vi "front_panel_new.vi"() -> ()   [LabVIEW 2026]
uses:
  <vilib>/userDefined/High Color/IMAQdx.ctl
  <vilib>/vision/driver/NI_Vision_Acquisition_Software.lvlib
  <resource>/objmgr/imaqdx.rc
panel:
  in  "Space":bool
  in  "Ready to Speak":bool
  in  "Speak":bool
  out "Text":string
  in  "Hand":bool
  in  "Next_letter":bool
  in  "Input":bool
  in  "Filename":string
  out "Image":T1(plugin-control)
  out "Prediction":string
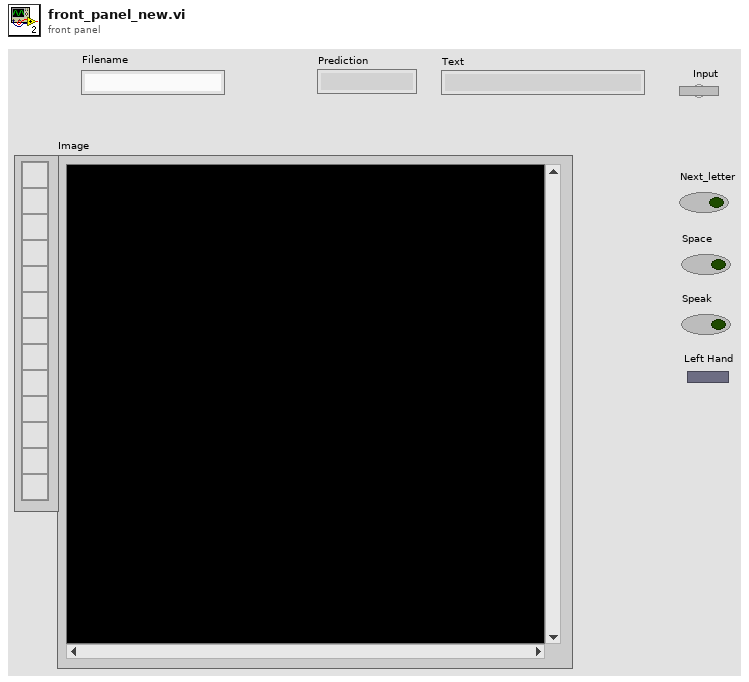
[diagram p1: front panel]
types:
  T1 = typedef "IMAQ Image.ctl" = refnum<image>
  T2 = typedef "IMAQdx.ctl" = refnum<k21>
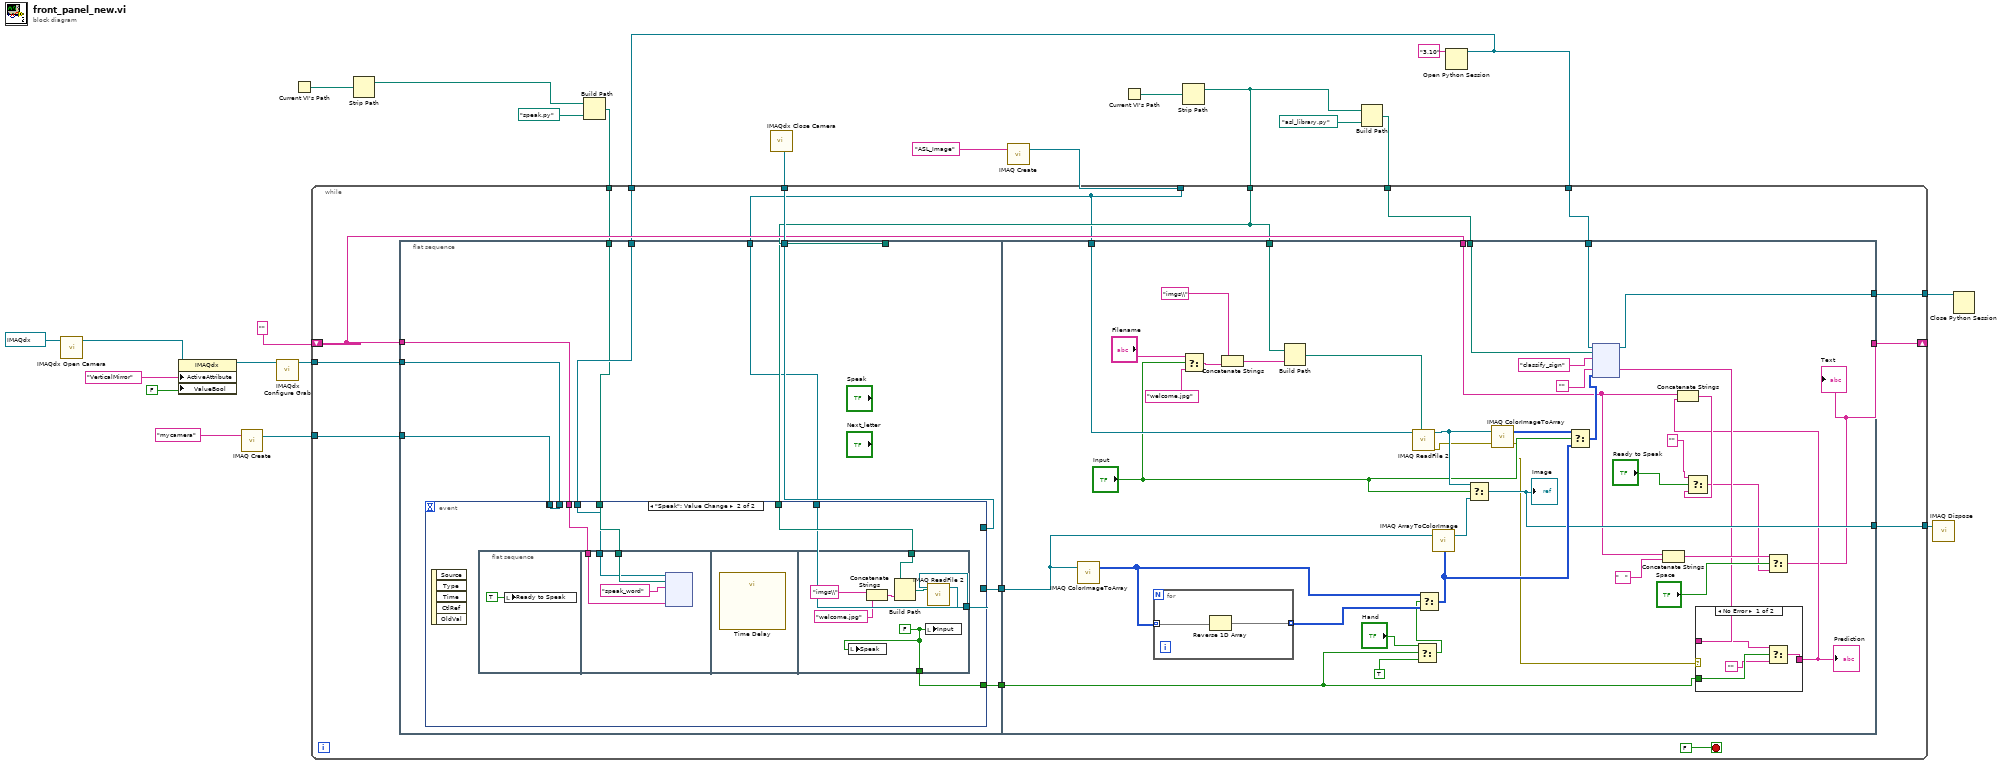
[diagram p0: block diagram]
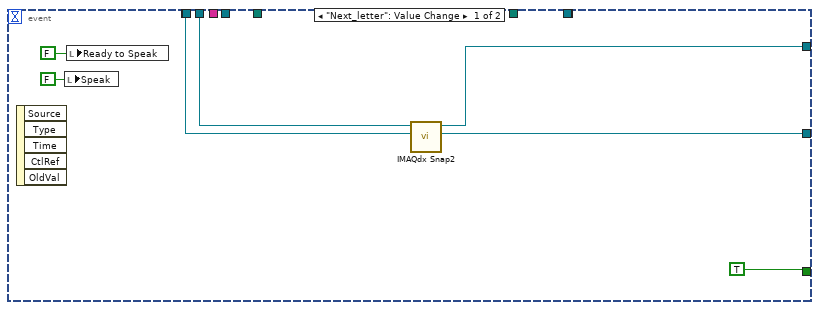
[diagram p2: hidden frame]
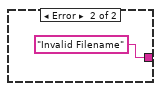
[diagram p3: hidden frame]
diagram:
  n1 = call <vilib>:"IMAQdx Open Camera.vi"("Session In"=T2 "cam0") -> ("Session Out"=w23:T2)  [unwired: 9 in, 1 out]
  n2 = property class="IMAQdx"(reference=w23, "ActiveAttribute"="VerticalMirror", "ValueBool"=FALSE) -> (reference out=w24:T2)  [unwired: 1 in, 1 out]
  n3 = call "IMAQ Create"("Image Name"="mycamera") -> ("New Image"=w17:T1)  [unwired: 4 in, 1 out]
  n4 = call <vilib>:"IMAQdx Configure Grab.vi"("Session In"=w24) -> ("Session Out"=w19:T2)  [unwired: 9 in, 1 out]
  n5 = Current VI's Path() -> (path=w4:path)
  n6 = Strip Path(path=w4) -> (stripped path=w2:path)  [unwired: 1 out]
  n7 = Build Path(base path=w2, name or relative path=path "speak.py" ("module path")) -> (appended path=w1:path)
  n8 = call "IMAQ Create"("Image Name"="ASL_Image") -> ("New Image"=w7:T1)  [unwired: 4 in, 1 out]
  n9 = Current VI's Path() -> (path=w12:path)
  n10 = Strip Path(path=w12) -> (stripped path=w9:path)  [unwired: 1 out]
  n11 = Build Path(base path=w9, name or relative path=path "asl_library.py" ("module path")) -> (appended path=w10:path)
  n12 = Open Python Session(python version="3.10" ("Python version")) -> (session out=w5:refnum<k35>)  [unwired: 2 in, 1 out]
  n13 = while {
    tunnel: w19 -> [w39]
    tunnel: w17 -> [w38]
    tunnel: [w37] -> w16
    tunnel: [w36] -> w15
    tunnel: [w35] -> w14
    tunnel: w5 -> [w34]
    tunnel: w10 -> [w33]
    tunnel: w9 -> [w28]
    tunnel: w7 -> [w27]
    shift-right: [w31] -> _
    shift-left: "" -> [w30]
    tunnel: w5 -> [w29]
    tunnel: w1 -> [w26]
    stop <- FALSE stop-if-true
    n14 = flat-sequence {
      tunnel: [w50] -> w40
      tunnel: w39 -> [w49]
      tunnel: w38 -> [w48]
      tunnel: [w47] -> w35
      tunnel: w30 -> [w46]
      tunnel: w29 -> [w45]
      tunnel: w28 -> [w44]
      tunnel: w27 -> [w43]
      tunnel: w26 -> [w42]
      tunnel: [w41] -> w25
      tunnel: w40 -> [w114]
      tunnel: [w106] -> w37
      tunnel: [w105] -> w36
      tunnel: w34 -> [w104]
      tunnel: w33 -> [w103]
      tunnel: w28 -> [w102]
      tunnel: w27 -> [w101]
      tunnel: w30 -> [w94]
      tunnel: [w83] -> w31
      tunnel: w25 -> [w86]
      frame #0 {
        n15 = event shown="[1] \"Speak\": Value Change" {
          selector: _ -> [_ _]
          dyn-events: _ -> [_ _]
          timeout: _ -> [_ _]
          tunnel: [w58 w62] -> w50
          tunnel: [w57 _] -> w47
          tunnel: w49 -> [w56 w66]
          tunnel: w48 -> [w55 _]
          tunnel: w46 -> [_ w60]
          tunnel: [_ w66] -> _
          tunnel: w45 -> [_ w61]
          tunnel: w44 -> [_ w64]
          tunnel: w43 -> [w52 w63]
          tunnel: w42 -> [_ w65]
          tunnel: [w52 _] -> _
          tunnel: [TRUE ("Input") w59] -> w41
          event "Next_letter": Value Change {
            n16 = event-data() -> ()  [unwired: 1 in, 5 out]
            n17 = local write "Speak"(FALSE ("Speak")) -> ()
            n18 = local write "Ready to Speak"(FALSE ("Ready_to_Speak")) -> ()
            n19 = call <vilib>:"IMAQdx Snap2.vi"("Image In"=w55, "Session In"=w56) -> ("Image Out"=w58:T1, "Session Out"=w57:T2)  [unwired: 7 in, 1 out]
          }
          event "Speak": Value Change {
            n20 = event-data() -> ()  [unwired: 1 in, 5 out]
            n21 = flat-sequence {
              tunnel: w65 -> [w71]
              tunnel: w60 -> [w69]
              tunnel: w61 -> [w68]
              tunnel: w64 -> [w75]
              tunnel: w63 -> [w74]
              tunnel: [w73] -> w62
              tunnel: [w72] -> w59
              frame #0 {
                n22 = local write "Ready to Speak"(TRUE ("Ready_to_Speak")) -> ()
              }
              frame #1 {
                n23 = node(w68, w71, "speak_word" ("function name"), w69) -> ()  [unwired: 4 in, 4 out]
              }
              frame #2 {
                n24 = call "Time Delay"() -> ()  [unwired: 11 in, 1 out]
              }
              frame #3 {
                w72 = FALSE ("Input")
                n25 = local write "Speak"(w72) -> ()
                n26 = Concatenate Strings("imgs\\" ("string"), "welcome.jpg" ("string")) -> (w78:string)
                n27 = Build Path(base path=w75, name or relative path=w78) -> (appended path=w79:path)
                n28 = local write "Input"(w72) -> ()
                n29 = call "IMAQ ReadFile 2"("File Path"=w79, "Image"=w74) -> ("Image Out"=w73:T1)  [unwired: 5 in, 4 out]
              }
            }
          }
        }
      }
      frame #1 {
        n30 = call "IMAQ ColorImageToArray"("Image"=w114) -> ("Image Pixels (U32)"=w108:u32[][])  [unwired: 3 in, 2 out]
        n31 = for {
          tunnel: w108 -> [w126] mode=indexing
          tunnel: [w125] -> w107 mode=indexing
          n32 = Reverse 1D Array(array=w126) -> (reversed array=w125:u32[])
        }
        n33 = Select(t="Filename", s="Input", f="welcome.jpg") -> (s? t:f=w93:string)
        n34 = Concatenate Strings("imgs\\" ("string"), w93) -> (w119:string)
        n35 = Build Path(base path=w102, name or relative path=w119) -> (appended path=w118:path)
        n36 = call "IMAQ ReadFile 2"("File Path"=w118, "Image"=w101) -> ("error out"=w89:errorcluster, "Image Out"=w113:T1)  [unwired: 5 in, 3 out]
        n37 = Select(t="Hand", s=w86, f=TRUE) -> (s? t:f=w85:bool)
        n38 = Select(t=w108, s=w85, f=w107) -> (s? t:f=w109:u32[][])
        n39 = call "IMAQ ArrayToColorImage"("Image Pixels (U32)"=w109, "Image"=w114) -> ("Image Out"=w112:T1)  [unwired: 3 in, 1 out]
        n40 = Select(t=w113, s="Input", f=w112) -> (s? t:f=w105:T1)
        "Image" <- w105
        n41 = call "IMAQ ColorImageToArray"("Image"=w113, "error in (no error)"=w89) -> ("Image Pixels (U32)"=w111:u32[][], "error out"=w88:errorcluster)  [unwired: 2 in, 1 out]
        n42 = Select(t=w111, s="Input", f=w109) -> (s? t:f=w110:u32[][])
        n43 = node(w104, w103, "classify_sign" ("function name"), "", w110) -> (w106:refnum<k35>, w87:string)  [unwired: 2 in, 3 out]
        n44 = Concatenate Strings(w94, "   " ("string")) -> (w96:string)
        n45 = case shown="No Error" w88 {
          tunnel: w86 -> [w123 _]
          tunnel: w87 -> [w122 _]
          tunnel: [w121 "Invalid Filename"] -> w84
          frame No Error {
            n46 = Select(t=w122, s=w123, f="") -> (s? t:f=w121:string)
          }
          frame Error {
          }
        }
        "Prediction" <- w84
        n47 = Concatenate Strings(w94, w84) -> (w97:string)
        n48 = Select(t="", s="Ready to Speak", f=w97) -> (s? t:f=w82:string)
        n49 = Select(t=w96, s="Space", f=w82) -> (s? t:f=w83:string)
        "Text" <- w83
      }
    }
  }
  n50 = call <vilib>:"IMAQdx Close Camera.vi"("Session In"=w14) -> ()  [unwired: 10 in, 1 out]
  n51 = call "IMAQ Dispose"("Image"=w15) -> ()  [unwired: 5 in, 1 out]
  n52 = Close Python Session(session in=w16) -> ()  [unwired: 1 in, 1 out]
